vi "dataDisplay.vi"(7 "data":i32, 9 "string data":string, 10 "string in":string, 11 "string type":string) -> (3 "str out":string)   [LabVIEW 2017]
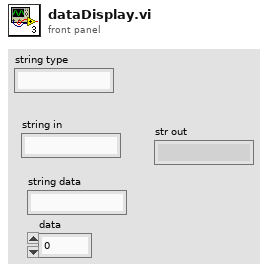
[diagram p1: front panel]
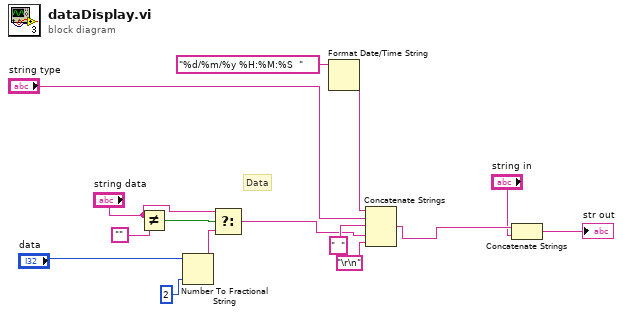
[diagram p0: block diagram]
diagram:
  # "Data"
  n1 = Not Equal?(x="string data", y="") -> (x != y?=w5:bool)
  n2 = Number To Fractional String(number="data", precision (6)=i16 2 ("width (-)")) -> (F-format string=w2:string)  [unwired: 2 in]
  n3 = Select(t="string data", s=w5, f=w2) -> (s? t:f=w3:string)
  n4 = Format Date/Time String(time format string (%c)="%d/%m/%y %H:%M:%S  ") -> (date/time string=w15:string)  [unwired: 2 in]
  n5 = Concatenate Strings(w15, "string type", "  " ("string"), w3, "\r\n") -> (w13:string)
  n6 = Concatenate Strings(w13, "string in") -> (→"str out":string)
